vi "Elapsed Time.vi"(10 "Reset?":bool) -> (2 "dt (ms)":u32)   [LabVIEW 2015]
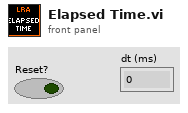
[diagram p1: front panel]
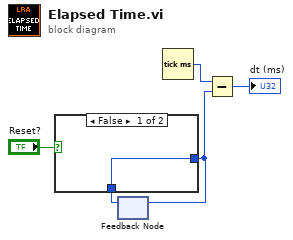
[diagram p0: block diagram]
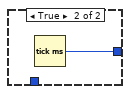
[diagram p2: hidden frame]
diagram:
  n1 = feedback #1() -> (w2:u32)  [unwired: 1 in]
  n2 = case shown="False" "Reset?" {
    tunnel: [w6 w7] -> w4
    tunnel: w2 -> [w6 _]
    frame False {
    }
    frame True {
      n3 = Tick Count (ms)() -> (millisecond timer value=w7:u32)
    }
  }
  n4 = feedback-in #1(w4) -> ()
  n5 = Tick Count (ms)() -> (millisecond timer value=w3:u32)
  n6 = Subtract(x=w3, y=w4) -> (x-y=→"dt (ms)":u32)
